vi "0-Save Image.vi"(8 "Error In":errorcluster, 11 "Image in":T1) -> (0 "Error Out":errorcluster)   [LabVIEW 2011]
uses:
  <vilib>/vision/Image Controls.llb/IMAQ Image.ctl
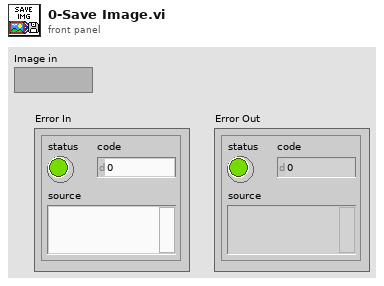
[diagram p1: front panel]
types:
  T1 = typedef "IMAQ Image.ctl" = refnum<image>
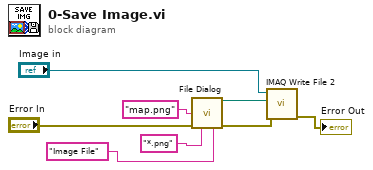
[diagram p0: block diagram]
diagram:
  n1 = call "File Dialog"("default name"="map.png", "error in"="Error In", "pattern (all files)"="*.png", "pattern label"="Image File") -> ("selected path"=w4:path, "error out"=w2:errorcluster)  [unwired: 3 in, 7 out]
  n2 = call-poly "IMAQ Write File 2"("error in (no error)"=w2, "File Path"=w4, "Image"="Image in") -> ("error out"=→"Error Out":errorcluster)  [unwired: 3 in, 5 out]
